vi "Actor Core.vi"(8 "error in":errorcluster, 11 "Signal Analysis in":refnum<class "Signal Analysis.lvclass">) -> (0 "error out":errorcluster, 3 "Actor out":refnum<class "Actor.lvclass">)   [LabVIEW 2020, in "Signal Analysis.lvlib" / "Signal Analysis.lvclass"]
doc: "<p>(<strong>Filename</strong>: <span class=\"dnl\">Actor Framework.lvlib:Actor.lvclass:Actor Core.vi</span>)</p>\n<p>Receives messages to the actor, reacts to them, and initiates any error handling that may shut the actor down.</p>\n<p>Descendant classes may override this VI to append parallel tasks for the actor to complete while it handles messages. Overrides use the <a href=\"nihelplauncher://docs/csh?context=lvcore_glang_udclass\">Call Parent Class Method</a> node.</p>"
uses:
  Signal Analysis.lvclass
  <vilib>/ActorFramework/Actor/Actor.lvclass
  Helper Loop Message.ctl
  Helper Loop Type.ctl
  Signal Analysis.lvclass/Signal Analysis.ctl
  Primitive/Primitive/Primitive.lvclass
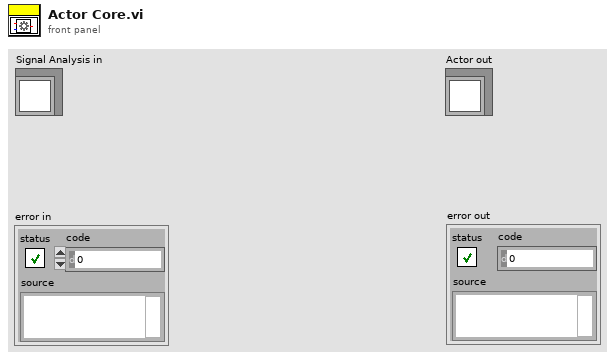
[diagram p1: front panel]
types:
  T1 = typedef "Signal Analysis.lvlib/Signal Analysis.lvclass/Helper Loop Message.ctl" = cluster{"Type":T2, "Payload":variant}
  T2 = typedef "Signal Analysis.lvlib/Signal Analysis.lvclass/Helper Loop Type.ctl" = enum16{"Process Data", "Set Batch Size", "Set Render Prio", "Close", "Set FFT Size"}
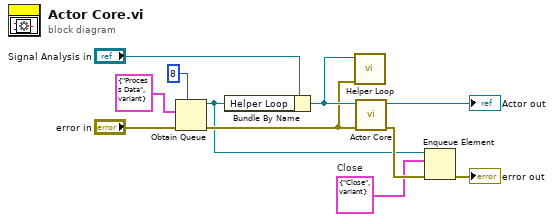
[diagram p0: block diagram]
diagram:
  w2 = T1 {"Type"=enum."Close", "Payload"=variant}  # Close
  n1 = Obtain Queue(max queue size (-1, unlimited)=8, element data type=T1 {"Type"=enum."Process Data", "Payload"=variant} ("Message"), error in (no error)="error in") -> (queue out=w3:refnum<queue>, error out=w7:errorcluster)  [unwired: 2 in, 1 out]
  n2 = Bundle By Name(cluster="Signal Analysis in", "Helper Loop"=w3) -> (w8:refnum<class "Signal Analysis.lvclass">)
  n3 = call "Helper Loop.vi"("error in (no error)"=w7, "Signal Analysis in"=w8) -> ()  [unwired: 10 in]
  n4 = call-parent "Actor Core.vi"("error in"=w7, "Actor in"=w8) -> ("error out"=w5:errorcluster, "Actor out"=→"Actor out":refnum<class "Actor.lvclass">)  [unwired: 8 in]
  n5 = Enqueue Element(queue=w3, element=w2, error in (no error)=w5) -> (error out=→"error out":errorcluster)  [unwired: 1 in, 2 out]
